vi "Find flexrio adapter module.vi"(8 "error in (no error)":errorcluster) -> (0 "error out":errorcluster, 2 "Devices & Chassis:Provides Link Name":string, 3 "NI 5772 adapter present ?":bool)   [LabVIEW 2020]
uses:
  <vilib>/nisyscfg/Expert Info.ctl
  <vilib>/nisyscfg/nisyscfg.lvlib
  <resource>/objmgr/nicontrollersysapi.rc
panel:
  out "Devices & Chassis:Slot Number":i32
  out "FlexRIO module name":string
  out "FlexRIO:Device Status":u32(ring) items=["Normal", "Thermal Shutdown", "Power Shutdown", "Firmware Update Needed", "Internal Error", "Fan Slowed", "Fan Stopped", "PLL Loss of Lock", "USB Over Current"]
  out "FlexRIO:Device Family":u32(ring) items=["Unknown", "PXIe-484X", "PXI-795X", "PXIe-796X", "PXIe-797X", "NI-793X", "PXIe-798X"]
  out "FlexRIO:Is Adapter Module":bool
  out "Supported Experts":T1[](array[typedef])
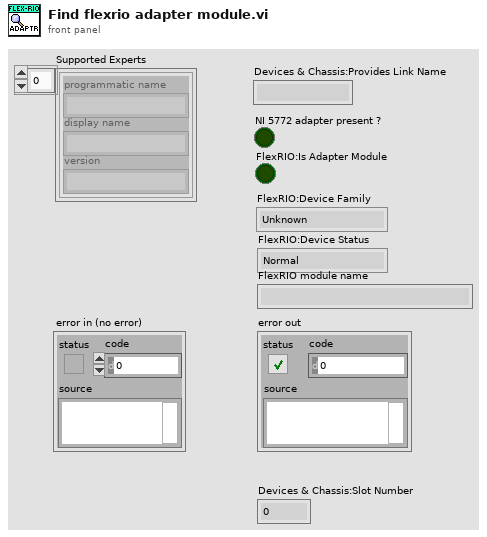
[diagram p1: front panel]
types:
  T1 = typedef "nisyscfg.lvlib/Expert Info.ctl" = cluster{"programmatic name":string, "display name":string, "version":string}
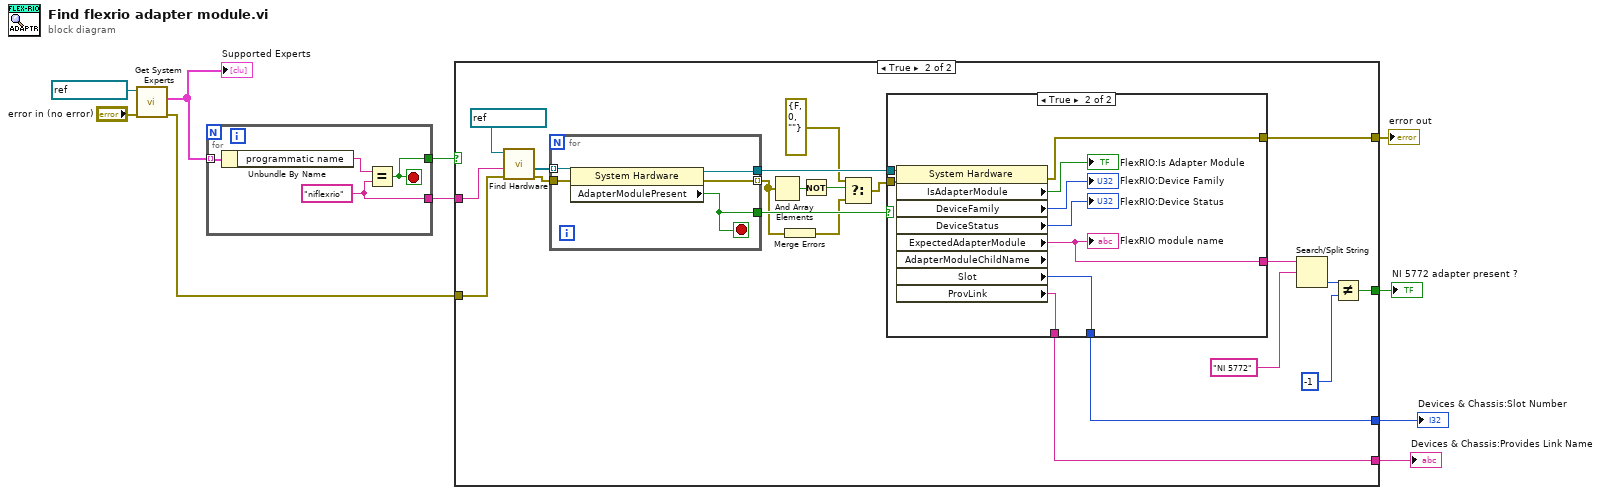
[diagram p0: block diagram]
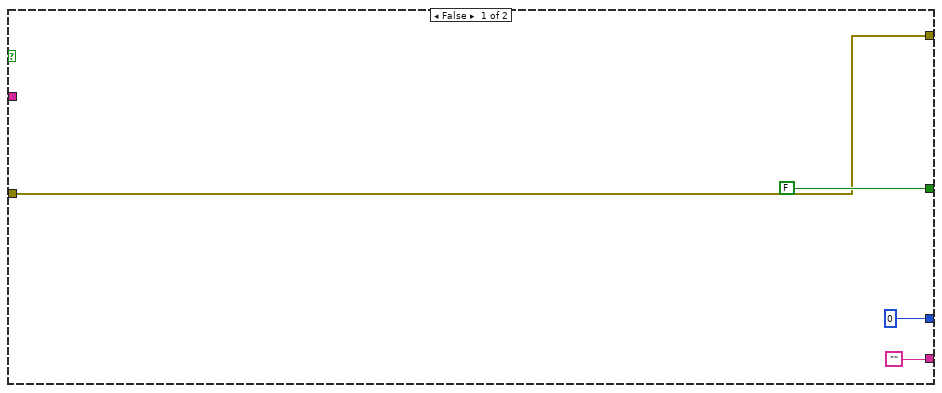
[diagram p2: hidden frame]
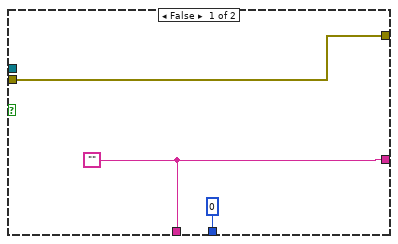
[diagram p3: hidden frame]
diagram:
  n1 = call <vilib>:"Get System Experts.vi"("error in (no error)"="error in (no error)", "Session in"=refnum<k21> "localhost") -> ("error out"=w4:errorcluster, "Supported Experts"=w9:T1[])  [unwired: 7 in, 1 out]
  "Supported Experts" <- w9
  n2 = for {
    tunnel: w9 -> [w14] mode=indexing
    tunnel: [w12] -> w7
    tunnel: [w11] -> w8
    stop <- w11 stop-if-true
    w12 = "niflexrio"
    n3 = Unbundle By Name(w14) -> ("programmatic name"=w13:string)
    n4 = Equal?(x=w13, y=w12) -> (x = y?=w11:bool)
  }
  n5 = case shown="True" w8 {
    tunnel: w7 -> [_ w38]
    tunnel: [FALSE w30] -> w6
    tunnel: w4 -> [w17 w29]
    tunnel: [w17 w27] -> w3
    tunnel: [0 ("Slot") w20] -> w2
    tunnel: ["" w19] -> w1
    frame False {
    }
    frame True {
      n6 = call <vilib>:"Find Hardware.vi"("error in (no error)"=w29, "Experts"=w38, "Session in"=refnum<k21> "localhost") -> ("error out"=w28:errorcluster, "Resources out"=w37:refnum<k20>[])  [unwired: 5 in, 2 out]
      n7 = for {
        tunnel: w37 -> [w56] mode=indexing
        tunnel: [w55] -> w36
        tunnel: [w54] -> w35
        tunnel: w28 -> [w53]
        tunnel: [w52] -> w23 mode=indexing
        stop <- w54 stop-if-true
        n8 = property class="System Hardware"(reference=w56, error in=w53) -> (reference out=w55:refnum<k20>, error out=w52:errorcluster, "AdapterModulePresent"=w54:bool)
      }
      n9 = And Array Elements(Boolean array=w23) -> (logical AND=w26:bool)
      n10 = Merge Errors(w23) -> (w22:errorcluster)
      n11 = Not(x=w26) -> (.not. x?=w25:bool)
      n12 = Select(t=errorcluster {"status"=FALSE, "code"=0, "source"=""} ("error constant"), s=w25, f=w22) -> (s? t:f=w21:errorcluster)
      n13 = case shown="True" w35 {
        tunnel: w36 -> [_ w51]
        tunnel: [w40 w47] -> w34
        tunnel: w21 -> [w42 w45]
        tunnel: [w42 w46] -> w27
        tunnel: [0 ("Slot") w44] -> w20
        tunnel: [w40 w43] -> w19
        frame False {
          w40 = ""
        }
        frame True {
          n14 = property class="System Hardware" props=["IsAdapterModule", "DeviceFamily", "DeviceStatus", "ExpectedAdapterModule", "AdapterModuleChildName", "Slot", "ProvLink"](reference=w51, error in=w45) -> (error out=w46:errorcluster, "IsAdapterModule"=→"FlexRIO:Is Adapter Module":bool, "DeviceFamily"=→"FlexRIO:Device Family":u32, "DeviceStatus"=→"FlexRIO:Device Status":u32, "ExpectedAdapterModule"=w47:string, "Slot"=w44:i32, "ProvLink"=w43:string)  [unwired: 2 out]
          "FlexRIO module name" <- w47
        }
      }
      n15 = Search/Split String(string=w34, search string/char (-)="NI 5772") -> (offset of match=w32:i32)  [unwired: 1 in, 2 out]
      n16 = Not Equal?(x=w32, y=-1) -> (x != y?=w30:bool)
    }
  }
  "NI 5772 adapter present ?" <- w6
  "error out" <- w3
  "Devices & Chassis:Slot Number" <- w2
  "Devices & Chassis:Provides Link Name" <- w1
